vi "grab image.vi"(8 "ErrorIn":errorcluster, 9 "BuffNr 2":i16, 10 "BuffNr":i16, 11 "ph":u64) -> (0 "output image":u16[][](array[numeric]), 1 "error out":errorcluster, 2 "Buffer_Ready":bool, 3 "hout":u64)   [LabVIEW 2014]
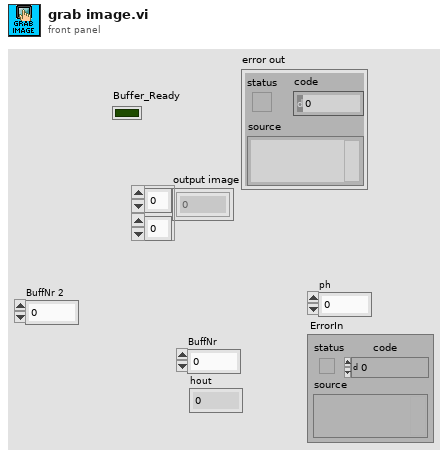
[diagram p1: front panel]
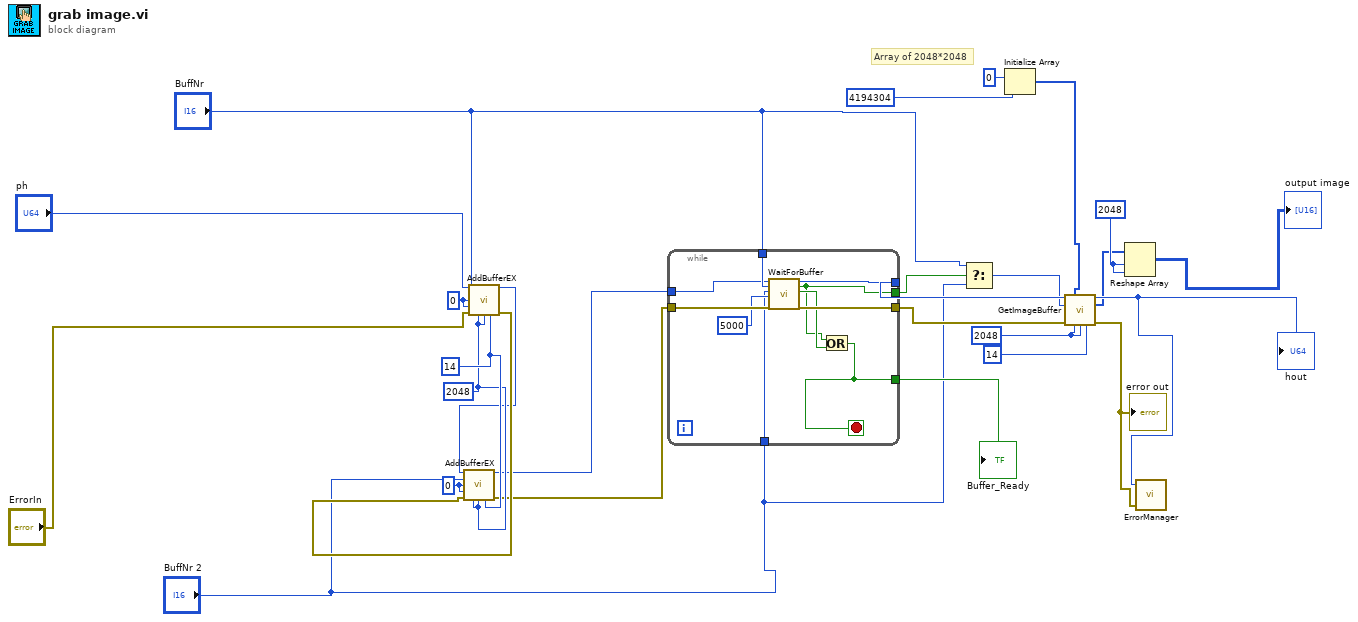
[diagram p0: block diagram]
diagram:
  w1 = u32 0 ("1stImage")
  w9 = u16 2048 ("yRes")
  w22 = u32 0 ("1stImage")
  w23 = 2048
  w18 = u16 2048
  w19 = u16 14
  # "Array of 2048*2048"
  n1 = call <userlib>:"AddBufferEX.vi"("ph"="ph", "BuffNr"="BuffNr", "1stImage"=w22, "LastImage"=w22, "error in (no error)"="ErrorIn", "XRes"=w18, "YRes"=w18, "BitPerPixel"=w19) -> ("hout"=w15:u64, "error out"=w17:errorcluster)  [unwired: 5 in, 1 out]
  n2 = call <userlib>:"AddBufferEX.vi"("ph"=w15, "BuffNr"="BuffNr 2", "1stImage"=w1, "LastImage"=w1, "error in (no error)"=w17, "XRes"=w18, "YRes"=w18, "BitPerPixel"=w19) -> ("hout"=w14:u64, "error out"=w13:errorcluster)  [unwired: 5 in, 1 out]
  n3 = while {
    tunnel: w14 -> [w28]
    tunnel: w13 -> [w37]
    tunnel: [w35] -> w25
    tunnel: [w34] -> w24
    tunnel: "BuffNr" -> [w33]
    tunnel: [w30] -> w21
    tunnel: "BuffNr 2" -> [w32]
    tunnel: [w29] -> w2
    stop <- w30 stop-if-true
    n4 = call <userlib>:"WaitForBuffer.vi"("ph"=w28, "sBufNr"=w33, "sBufNr 2"=w32, "timeout"=u32 5000, "error in (no error)"=w37) -> ("hout"=w35:u64, "Buffer_Ready"=w29:bool, "Buffer_Ready 2"=w31:bool, "error out"=w34:errorcluster)  [unwired: 10 in, 1 out]
    n5 = Or(x=w29, y=w31) -> (x .or. y?=w30:bool)
  }
  "Buffer_Ready" <- w21
  n6 = Select(t="BuffNr", s=w2, f="BuffNr 2") -> (s? t:f=w10:i16)
  n7 = Initialize Array(i16 0 ("element"), 4194304 ("dimension size")) -> (w5:i16[])
  n8 = call <userlib>:"GetImageBuffer.vi"("ph"=w25, "BuffIn"=w5, "BuffNr"=w10, "error in (no error)"=w24, "xRes"=w9, "yRes"=w9, "Bitresolution"=u16 14) -> ("hout"=w7:u64, "BuffOut"=w4:u16[], "error out"=w6:errorcluster)  [unwired: 5 in, 1 out]
  "hout" <- w7
  "error out" <- w6
  n9 = Reshape Array(w4, w23, w23) -> (→"output image":u16[][])
  n10 = call <userlib>:"ErrorManager.vi"("ErrorIn"=w6, "ErrorCode"=w7) -> ()  [unwired: 3 in, 1 out]
